vi "Create New VI.vi"   [LabVIEW 2017]
doc: "Creates new VI from BenjaminR's VI Template."
types:
  T1 = enum32{"Invalid", "Standard", "Closed", "Hidden", "Minimized", "Maximized"}
  T2 = enum32{"invalid VI type", "Standard VI", "Control VI", "Global VI", "Polymorphic VI", "Configuration VI", "SubSystem", "Facade VI", "Method VI", "Statechart Diagram VI"}
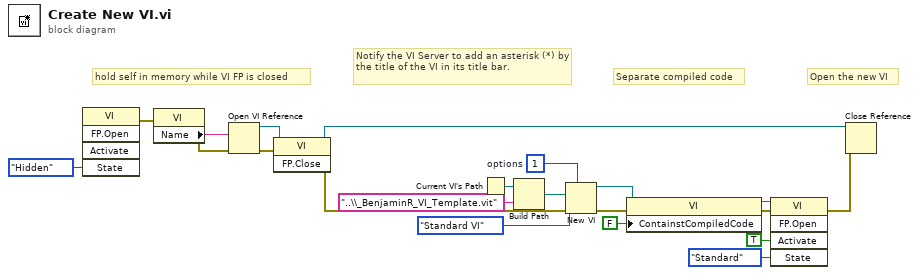
[diagram p0: block diagram]
diagram:
  w6 = u32 1  # options
  # "Open the new VI"
  # "Separate compiled code"
  # "Notify the VI Server to add an asterisk (*) by the title of the VI in its title bar."
  # "hold self in memory while VI FP is closed"
  n1 = invoke class="VI" method="FP.Open"("State"=T1."Hidden") -> (error out=w13:errorcluster)  [unwired: 4 in, 4 out]
  n2 = property class="VI"(error in=w13) -> (error out=w14:errorcluster, "Name"=w18:string)  [unwired: 1 in, 1 out]
  n3 = Open VI Reference(vi path=w18, error in (no error)=w14) -> (vi reference=w17:refnum<vi>, error out=w16:errorcluster)  [unwired: 4 in]
  n4 = invoke class="VI" method="FP.Close"(reference=w17, error in=w16) -> (reference out=w11:refnum<vi>, error out=w12:errorcluster)  [unwired: 1 in, 1 out]
  n5 = Current VI's Path() -> (path=w21:path)
  n6 = Build Path(base path=w21, name or relative path="..\\_BenjaminR_VI_Template.vit") -> (appended path=w19:path)
  n7 = New VI(7:w6, 8:w12, 9:T2."Standard VI" ("vi type (standard vi)"), 10:w19) -> (0:w9:errorcluster, 3:w8:refnum<vi>)  [unwired: 3 in]
  n8 = property class="VI"(reference=w8, error in=w9, "ContainstCompiledCode"=FALSE ("Contains Compiled Code")) -> (reference out=w5:refnum<vi>, error out=w4:errorcluster)
  n9 = invoke class="VI" method="FP.Open"(reference=w5, error in=w4, "Activate"=TRUE ("Activate?"), "State"=T1."Standard") -> (error out=w3:errorcluster)  [unwired: 1 in, 4 out]
  n10 = Close Reference(reference=w11, error in (no error)=w3) -> ()  [unwired: 1 out]
